vi "Read from Network.vi"() -> ()   [LabVIEW 2015]
uses:
  <vilib>/Platform/storage/Storage.llb/usiSequenceRepresentation.ctl
  <vilib>/Platform/storage/Storage.llb/usiOverwriteOptions.ctl
  <vilib>/Platform/storage/lvStorage.llb/_defaultFilePath.vi
  <vilib>/Platform/storage/lvStorage.llb/_openStorageWithRootAutoDetect.vi
  <vilib>/Platform/storage/lvStorage.llb/xStorage/xStorageSupp/ErrorOut.vi
  <vilib>/Platform/storage/lvStorage.llb/_createOrGetExplicitChildObject.vi
  <vilib>/Platform/storage/lvStorage.llb/_createOrGetByNameExplicitChildObject.vi
  <vilib>/Platform/storage/lvStorage.llb/__saveStringChannel.vi
  <vilib>/Platform/storage/Storage.llb/Get Object Info.vi
  <vilib>/Platform/storage/Storage.llb/__closeStorageFromObject.vi
  <vilib>/Platform/storage/lvStorage.llb/xStorage/Open Data Storage/Open Data Storage.xnode
  <vilib>/Platform/storage/lvStorage.llb/xStorage/Write Data/Write Data.xnode
  <vilib>/Platform/storage/lvStorage.llb/xStorage/Close Data Storage/Close Data Storage.xnode
panel:
  in  "stop":bool
  in  "Start":bool
  out "data out":u32[](array[numeric])
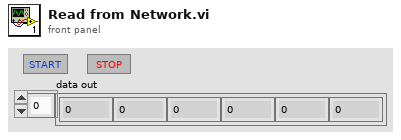
[diagram p1: front panel]
types:
  T1 = enum16{"open", "open or create", "create or replace", "create", "open (read only)"}
  T2 = enum16{"UPDATE", "READ", "QUERY", "CREATE CHILD", "CREATE", "CONNECT", "DISCONNECT"}
  T3 = typedef "usiOverwriteOptions.ctl" = enum16{"Append values", "Replace values at index", "Replace all values", "Append if timeline aligns"}
  T4 = typedef "usiSequenceRepresentation.ctl" = enum16{"explicit", "implicit"}
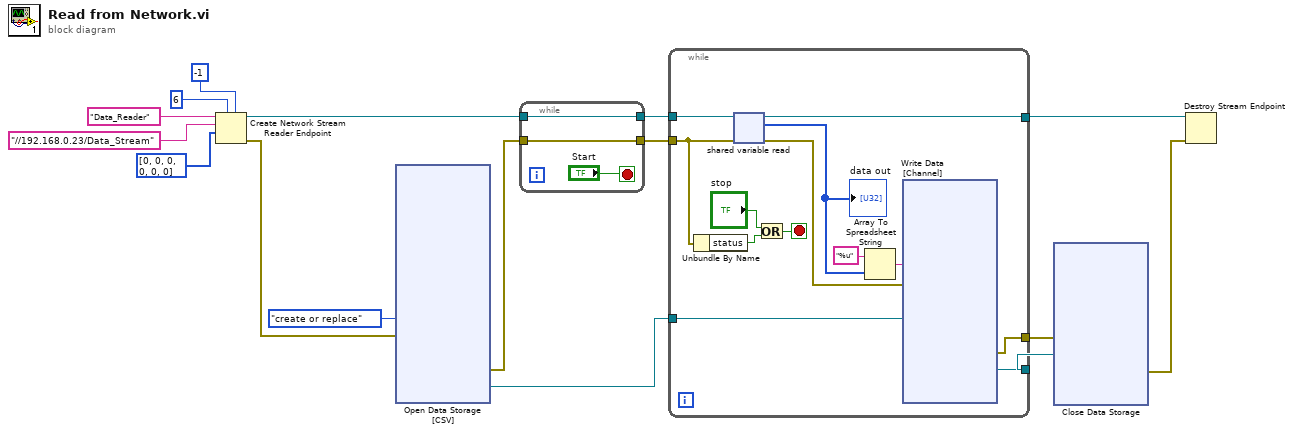
[diagram p0: block diagram]
diagram:
  n1 = Create Network Stream Reader Endpoint(5:-1 ("timeout in ms (-1)"), 7:6 ("writer buffer size"), 9:u32[] [0, 0, 0, 0, 0, 0], 10:"//192.168.0.23/Data_Stream" ("writer url"), 11:"Data_Reader" ("writer name")) -> (0:w6:errorcluster, 3:w10:refnum<k21>)  [unwired: 2 in]
  n2 = xnode "Open Data Storage\n[CSV]"("function (open:0)"=T1."create or replace", "error in (no error)"=w6) -> ("error out"=w3:errorcluster, "storage refnum (file)"=w5:refnum<k20>)  [unwired: 3 in, 1 out]
  n3 = while {
    tunnel: [w19] -> w9
    tunnel: w10 -> [w19]
    tunnel: w3 -> [w18]
    tunnel: [w18] -> w8
    stop <- "Start" stop-if-true
  }
  n4 = while {
    tunnel: [w31] -> w11
    tunnel: w9 -> [w32]
    tunnel: w8 -> [w26]
    tunnel: w5 -> [w30]
    tunnel: [w29] -> w4
    tunnel: [w27] -> w2
    stop <- w23 stop-if-true
    n5 = Unbundle By Name(w26) -> ("status"=w25:bool)
    n6 = shared-variable-read(w32, w26) -> (w31:refnum<k21>, w28:errorcluster, w22:u32[])  [unwired: 1 in, 1 out]
    "data out" <- w22
    n7 = Or(x="stop", y=w25) -> (x .or. y?=w23:bool)
    n8 = Array To Spreadsheet String(array=w22, 3:"%u" ("format string")) -> (spreadsheet string=w21:string)  [unwired: 1 in]
    n9 = xnode "Write Data\n[Channel]"("Signal"=w21, "error in"=w28, "storage refnum (file)"=w30) -> ("error out"=w27:errorcluster, "storage refnum (file) out"=w29:refnum<k20>)  [unwired: 2 in, 1 out]
  }
  n10 = xnode "Close Data Storage\n"("error in (no error)"=w2, "storage refnum (file)"=w4) -> ("error out"=w1:errorcluster)  [unwired: 1 out]
  n11 = Destroy Stream Endpoint(8:w1, 11:w11) -> ()  [unwired: 1 out]
